vi "TestColision.vi"() -> ()   [LabVIEW 2017]
uses:
  Display/Display_mods.ctl
  Spaceship/Spaceship_mods.ctl
  ManageMovableObjects/ManRef_mods.ctl
  Asteroid/Asteroid_data.ctl
  GameConfig/GameConfig_data.ctl
  <vilib>/Utility/inputDevices.llb/keyboardAcquire.vi
  <userlib>/_OpenG.lib/numeric/numeric.llb/Random Number Within Range - DBL__ogtk.vi
  <userlib>/_OpenG.lib/numeric/numeric.llb/Random Number Within Range - I32__ogtk.vi
  <vilib>/Utility/inputDevices.llb/closeKeyboard.vi
panel:
  in  "Add":bool
  out "error out":errorcluster
  in  "stop":bool
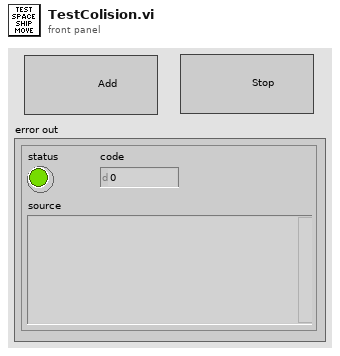
[diagram p1: front panel]
types:
  T1 = typedef "GameConfig_data.ctl" = cluster{"SpaceShip":cluster{"Angle":dbl, "SideLenght":dbl, "MaxLinearVeloc":dbl, "MaxAngularVeloc":dbl, "LinearAceleration":dbl, "AngularAceleration":dbl}, "Physics":cluster{"LinearDragFactor":dbl, "AngularDragFactor":dbl}, "Asteroids":cluster{"MaxSize":dbl, "MaxDivisions":i32, "MaxVeloc":dbl, "MinVeloc":dbl, "Fill":bool}, "Environment":cluster{"MaxAsteroids":i32, "TimeIncrement":dbl, "AsterProbCreation":dbl}, "Shots":cluster{"MinTimeShots":dbl, "ShotSize":dbl, "ShotSpeed":dbl}}
  T2 = typedef "ManRef_mods.ctl" = enum16{"Init", "NewAster", "MoveAll", "DestroyAster", "NewShoot", "DestroyShot", "CheckColision", "End"}
  T3 = typedef "Spaceship_mods.ctl" = enum16{"Init", "Move", "Rotate", "Translate", "GetData", "End"}
  T4 = typedef "Display_mods.ctl" = enum16{"Init", "GetBase", "DrawAster", "DrawShip", "DrawShoot", "Clear", "Close"}
  T5 = typedef "Asteroid_data.ctl" = cluster{"Veloc":dbl, "Direction":dbl, "Size":i32, "displayRef":refnum<vi>, "Max X":dbl, "Max Y":dbl, "Xpos":dbl, "Ypos":dbl, "ID":i32, "Config":T1}
  T6 = enum16{"0", "1", "2", "3", "4", "5", "6", "7", "8", "9", "A", "B", "C", "D", "E", "F", "G", "H", "I", "J", "K", "L", "M", "N", "O", "P", "Q", "R", "S", "T", "U", "V", "W", "X", "Y", "Z", "F1", "F2", "F3", "F4", "F5", "F6", "F7", "F8", "F9", "F10", "F11", "F12", "F13", "F14", "F15", "ADD", "BACK", "BACKSLASH", "CAPITAL", "COMMA", "DECIMAL", "DELETE", "DIVIDE", "DOWN", "END", "EQUALS", "ESCAPE", "GRAVE (`)", "HOME", "INSERT", "LBRACKET", "LCONTROL", "LEFT", "L ALT", "LSHIFT", "LWIN", "MINUS", "MULTIPLY", "NEXT", "NUMLOCK", "NUMPAD_0", "NUMPAD_1", "NUMPAD_2", "NUMPAD_3", "NUMPAD_4", "NUMPAD_5", "NUMPAD_6", "NUMPAD_7", "NUMPAD_8", "NUMPAD_9", "PAUSE", "PERIOD", "PRIOR (PG UP)", "RBRACKET", "RCONTROL", "RETURN", "RIGHT", "R ALT", "RSHIFT", "RWIN", "SCROLL", "SEMICOLON", "SLASH", "SPACE", "SUBTRACT", "TAB", "UP", "ENTER (num pad)", "' (quote)"}[]
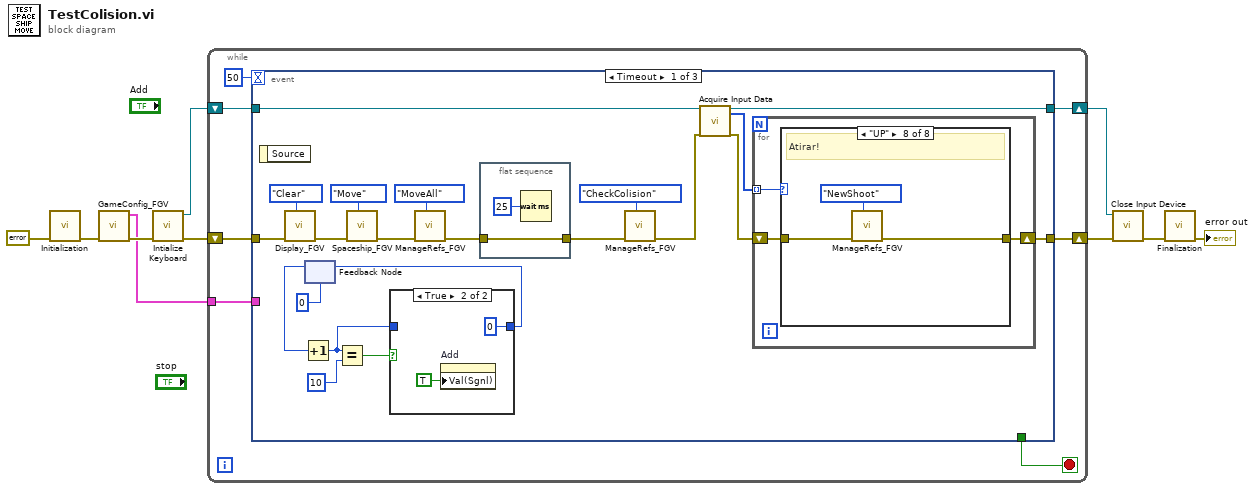
[diagram p0: block diagram]
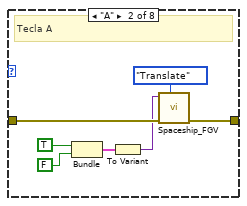
[diagram p4: hidden frame]
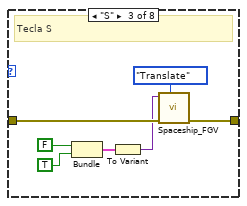
[diagram p5: hidden frame]
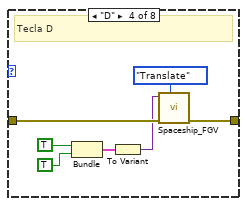
[diagram p6: hidden frame]
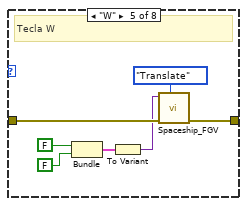
[diagram p7: hidden frame]
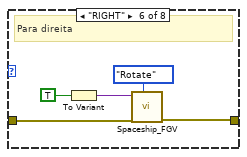
[diagram p8: hidden frame]
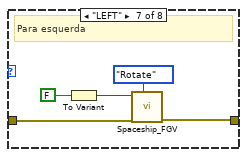
[diagram p9: hidden frame]
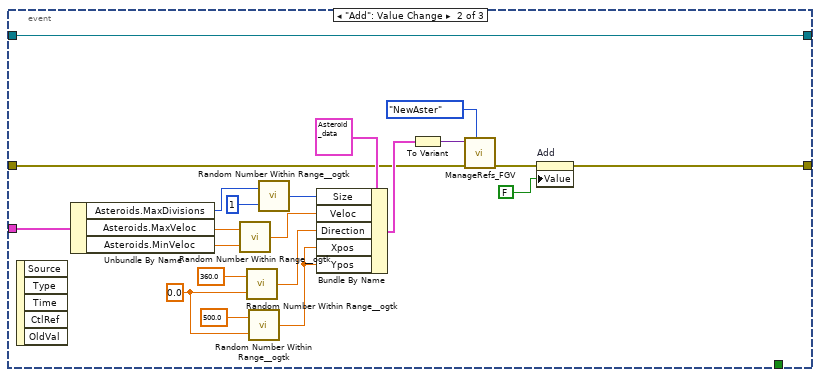
[diagram p10: hidden frame]
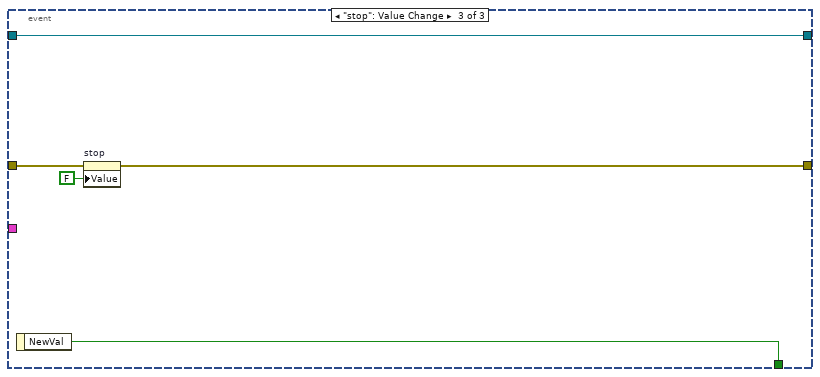
[diagram p11: hidden frame]
diagram:
  n1 = call "Initialization.vi"("error in"=errorcluster {"status"=FALSE, "code"=0, "source"=""}) -> ("error out"=w3:errorcluster)  [unwired: 10 in]
  n2 = call "GameConfig_FGV.vi"("error in"=w3) -> ("error out"=w2:errorcluster, "Config"=w1:T1)  [unwired: 9 in]
  n3 = call <vilib>:"Intialize Keyboard.vi"("error in (no error)"=w2) -> ("error out"=w8:errorcluster, "device ID"=w7:refnum<k1>)  [unwired: 9 in]
  n4 = while {
    shift-right: [w16] -> w6
    shift-left: w8 -> [w17]
    shift-right: [w12] -> w4
    shift-left: w7 -> [w13]
    tunnel: w1 -> [w11]
    stop <- w14 stop-if-true
    n5 = event shown="[0] Timeout" {
      selector: _ -> [_ _ _]
      dyn-events: _ -> [_ _ _]
      timeout: 50 -> [_ _ _]
      tunnel: w17 -> [w37 w93 w112]
      tunnel: [w32 w92 w111] -> w16
      tunnel: [_ _ w114] -> w14
      tunnel: w13 -> [w34 w89 w110]
      tunnel: [w33 w89 w110] -> w12
      tunnel: w11 -> [_ w90 _]
      event Timeout {
        n6 = event-data() -> ()  [unwired: 1 in, 1 out]
        n7 = call "Display_FGV.vi"("Display_mods"=Display_mods."Clear", "error in"=w37) -> ("error out"=w36:errorcluster)  [unwired: 8 in, 1 out]
        n8 = feedback #1(0) -> (w28:i32)
        n9 = Increment(x=w28) -> (x+1=w23:i32)
        n10 = Equal?(x=w23, y=10) -> (x = y?=w25:bool)
        n11 = call "Spaceship_FGV.vi"("Spaceship_mods"=Spaceship_mods."Move", "error in"=w36) -> ("error out"=w30:errorcluster)  [unwired: 8 in, 1 out]
        n12 = case shown="True" w25 {
          tunnel: [w41 0] -> w24
          tunnel: w23 -> [w41 _]
          frame False {
          }
          frame True {
            n13 = property on="Add" class="Bool (strict)"("Val(Sgnl)"=TRUE ("Value (Signaling)")) -> ()  [unwired: 2 in, 2 out]
          }
        }
        n14 = feedback-in #1(w24) -> ()
        n15 = call "ManageRefs_FGV.vi"("ManRef_mods"=ManRef_mods."MoveAll", "error in"=w30) -> ("error out"=w20:errorcluster)  [unwired: 9 in]
        n16 = flat-sequence {
          tunnel: w20 -> [w39]
          tunnel: [w39] -> w19
          frame #0 {
            n17 = Wait (ms)(milliseconds to wait=u32 25) -> ()  [unwired: 1 out]
          }
        }
        n18 = call "ManageRefs_FGV.vi"("ManRef_mods"=ManRef_mods."CheckColision", "error in"=w19) -> ("error out"=w21:errorcluster)  [unwired: 9 in]
        n19 = call-poly <vilib>:"Acquire Input Data.vi"("device ID"=w34, "error in (no error)"=w21) -> ("device ID"=w33:refnum<k1>, "keys pressed"=w31:T6, "error out"=w18:errorcluster)  [unwired: 15 in]
        n20 = for {
          shift-right: [w45] -> w32
          shift-left: w18 -> [w46]
          tunnel: w31 -> [w44] mode=indexing
          n21 = case shown="\"UP\"" w44 {
            tunnel: w46 -> [w47 w53 w60 w67 w74 w79 w84 w87]
            tunnel: [w47 w52 w59 w66 w73 w78 w83 w86] -> w45
            frame "0", Default {
            }
            frame "A" {
              # "Tecla A"
              n22 = Bundle("stop"=TRUE, "stop"=FALSE) -> (w51:cluster{"stop":bool, "stop":bool})  [unwired: 1 in]
              n23 = To Variant(anything=w51) -> (Variant=w50:variant)
              n24 = call "Spaceship_FGV.vi"("Spaceship_mods"=Spaceship_mods."Translate", "error in"=w53, "DataIn"=w50) -> ("error out"=w52:errorcluster)  [unwired: 7 in, 1 out]
            }
            frame "S" {
              # "Tecla S"
              n25 = Bundle("stop"=FALSE, "stop"=TRUE) -> (w58:cluster{"stop":bool, "stop":bool})  [unwired: 1 in]
              n26 = To Variant(anything=w58) -> (Variant=w57:variant)
              n27 = call "Spaceship_FGV.vi"("Spaceship_mods"=Spaceship_mods."Translate", "error in"=w60, "DataIn"=w57) -> ("error out"=w59:errorcluster)  [unwired: 7 in, 1 out]
            }
            frame "D" {
              # "Tecla D"
              n28 = Bundle("stop"=TRUE, "stop"=TRUE) -> (w65:cluster{"stop":bool, "stop":bool})  [unwired: 1 in]
              n29 = To Variant(anything=w65) -> (Variant=w64:variant)
              n30 = call "Spaceship_FGV.vi"("Spaceship_mods"=Spaceship_mods."Translate", "error in"=w67, "DataIn"=w64) -> ("error out"=w66:errorcluster)  [unwired: 7 in, 1 out]
            }
            frame "W" {
              # "Tecla W"
              n31 = Bundle("stop"=FALSE, "stop"=FALSE) -> (w72:cluster{"stop":bool, "stop":bool})  [unwired: 1 in]
              n32 = To Variant(anything=w72) -> (Variant=w71:variant)
              n33 = call "Spaceship_FGV.vi"("Spaceship_mods"=Spaceship_mods."Translate", "error in"=w74, "DataIn"=w71) -> ("error out"=w73:errorcluster)  [unwired: 7 in, 1 out]
            }
            frame "RIGHT" {
              # "Para direita"
              n34 = To Variant(anything=TRUE ("stop")) -> (Variant=w77:variant)
              n35 = call "Spaceship_FGV.vi"("Spaceship_mods"=Spaceship_mods."Rotate", "error in"=w79, "DataIn"=w77) -> ("error out"=w78:errorcluster)  [unwired: 7 in, 1 out]
            }
            frame "LEFT" {
              # "Para esquerda"
              n36 = To Variant(anything=FALSE ("stop")) -> (Variant=w82:variant)
              n37 = call "Spaceship_FGV.vi"("Spaceship_mods"=Spaceship_mods."Rotate", "error in"=w84, "DataIn"=w82) -> ("error out"=w83:errorcluster)  [unwired: 7 in, 1 out]
            }
            frame "UP" {
              # "Atirar!"
              n38 = call "ManageRefs_FGV.vi"("ManRef_mods"=ManRef_mods."NewShoot", "error in"=w87) -> ("error out"=w86:errorcluster)  [unwired: 9 in]
            }
          }
        }
      }
      event "Add": Value Change {
        w99 = 0.0 ("Low")
        n39 = event-data() -> ()  [unwired: 1 in, 5 out]
        n40 = Unbundle By Name(w90) -> ("Asteroids.MaxDivisions"=w105:i32, "Asteroids.MaxVeloc"=w103:dbl, "Asteroids.MinVeloc"=w104:dbl)
        n41 = call-poly <userlib>:"Random Number Within Range__ogtk.vi"("High"=w103, "Low"=w104) -> ("Random Number"=w107:dbl)  [unwired: 3 in]
        n42 = call-poly <userlib>:"Random Number Within Range__ogtk.vi"("High"=360.0, "Low"=w99) -> ("Random Number"=w108:dbl)  [unwired: 3 in]
        n43 = call-poly <userlib>:"Random Number Within Range__ogtk.vi"("High"=500.0, "Low"=w99) -> ("Random Number"=w91:dbl)  [unwired: 3 in]
        n44 = call-poly <userlib>:"Random Number Within Range__ogtk.vi"("High"=w105, "Low"=1) -> ("Random Number"=w106:i32)  [unwired: 3 in]
        n45 = Bundle By Name(cluster=T5 {"Veloc"=100.0, "Direction"=0.0, "Size"=3, "displayRef"=refnum, "Max X"=0.0, "Max Y"=0.0, "Xpos"=0.0, "Ypos"=150.0, "ID"=0, "Config"={"SpaceShip"={"Angle"=30.0, "SideLenght"=2.0, "MaxLinearVeloc"=10.0, "MaxAngularVeloc"=10.0, "LinearAceleration"=1.0, "AngularAceleration"=1.0}, "Physics"={"LinearDragFactor"=1.0, "AngularDragFactor"=1.0}, "Asteroids"={"MaxSize"=6.0, "MaxDivisions"=3, "MaxVeloc"=8.0, "MinVeloc"=1.0, "Fill"=FALSE}, "Environment"={"MaxAsteroids"=10, "TimeIncrement"=0.1, "AsterProbCreation"=0.1}, "Shots"={"MinTimeShots"=10.0, "ShotSize"=0.1, "ShotSpeed"=0.1}}} ("AsteroidData"), "Size"=w106, "Veloc"=w107, "Direction"=w108, "Xpos"=w91, "Ypos"=w91) -> (w109:T5)
        n46 = To Variant(anything=w109) -> (Variant=w101:variant)
        n47 = call "ManageRefs_FGV.vi"("ManRef_mods"=ManRef_mods."NewAster", "error in"=w93, "DataIn"=w101) -> ("error out"=w102:errorcluster)  [unwired: 8 in]
        n48 = property on="Add" class="Bool (strict)"(error in=w102, "Value"=FALSE ("Add")) -> (error out=w92:errorcluster)  [unwired: 1 in, 1 out]
      }
      event "stop": Value Change {
        n49 = event-data() -> ("NewVal"=w114:bool)  [unwired: 1 in]
        n50 = property on="stop" class="Bool (strict)"(error in=w112, "Value"=FALSE ("Add")) -> (error out=w111:errorcluster)  [unwired: 1 in, 1 out]
      }
    }
  }
  n51 = call-poly <vilib>:"Close Input Device.vi"("error in (no error)"=w6, "device ID"=w4) -> ("error out"=w5:errorcluster)  [unwired: 8 in]
  n52 = call "Finalization.vi"("error in"=w5) -> ("error out"=→"error out":errorcluster)  [unwired: 10 in]
